vi "G#Interface_GetInstance.vi"(0 "reference in":refnum<class "G#Object.lvclass">, 5 "error in (no error)":errorcluster) -> (14 "reference out":refnum<class "G#Object.lvclass">, 15 "not a refnum?":bool, 16 "G#Object":refnum<class "G#Object.lvclass">, 19 "error out":errorcluster)   [LabVIEW 2020, in "G#Object.lvclass"]
doc: "Returns the instance to the G#Object that is wrapped behind the interface."
uses:
  <vilib>/addons/_AddQ/G#Object/G#Object.lvclass
panel:
  # "OBSOLETE!\nFor backward compability"
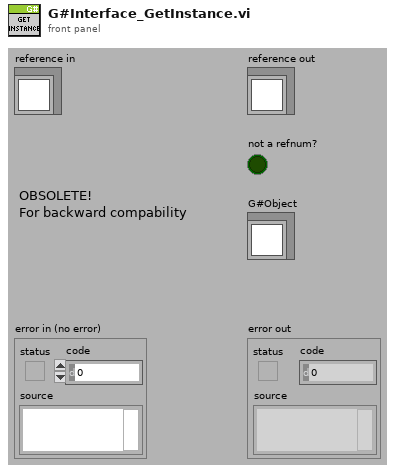
[diagram p1: front panel]
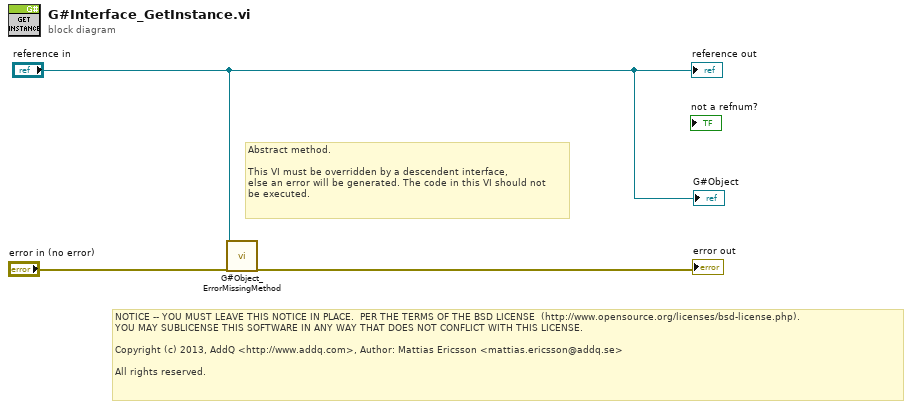
[diagram p0: block diagram]
diagram:
  # "Abstract method.\n\nThis VI must be overridden by a descendent interface,\nelse an error will be generated. The code in this VI should not\nbe executed."
  # "NOTICE -- YOU MUST LEAVE THIS NOTICE IN PLACE.  PER THE TERMS OF THE BSD LICENSE  (http://www.opensource.org/licenses/bsd-license.php).\nYOU MAY SUBLICENSE THIS SOFTWARE IN ANY WAY THAT DOES NOT CONFLICT WITH THIS LICENSE.\n\nCopyright (c) 2013, AddQ <http://www.addq.com>, Author: Mattias Ericsson <mattias.ericsson@addq.se>\n\nAll rights reserved."
  n1 = call-dynamic "G#Object_ErrorMissingMethod.vi"("reference in"="reference in", "error in (no error)"="error in (no error)") -> ("error out"=→"error out":errorcluster)  [unwired: 16 in, 1 out]
  "reference out" <- "reference in"
  "G#Object" <- "reference in"
